vi "HTML Hierarhy Add Leaf.vi"(8 "error in":errorcluster, 10 "id":string, 11 "label":string) -> (0 "error out":errorcluster)   [LabVIEW 2014, in "lvprj2html.lvlib"]
uses:
  lvprj2html.lvlib
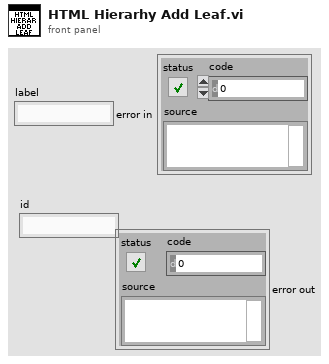
[diagram p1: front panel]
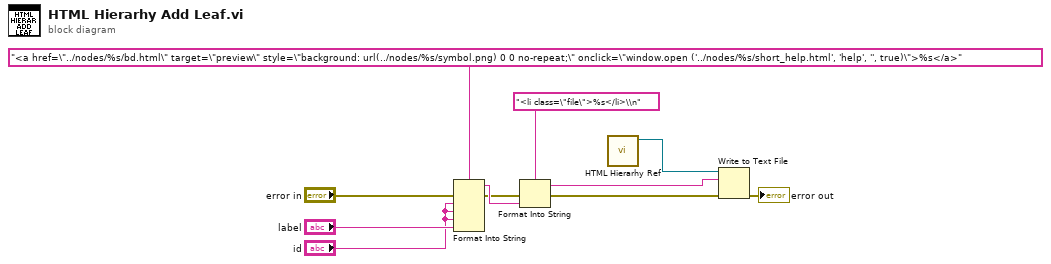
[diagram p0: block diagram]
diagram:
  n1 = Format Into String(format string="<a href=\"../nodes/%s/bd.html\" target=\"preview\" style=\"background: url(../nodes/%s/symbol.png) 0 0 no-repeat;\" onclick=\"window.open ('../nodes/%s/short_help.html', 'help', '', true)\">%s</a>" ("text"), error in="error in", "id", "id", "id", "label") -> (resulting string=w6:string, error out=w3:errorcluster)  [unwired: 1 in]
  n2 = Format Into String(format string="<li class=\"file\">%s</li>\\n" ("text"), error in=w3, w6) -> (resulting string=w5:string, error out=w2:errorcluster)  [unwired: 1 in]
  n3 = call "HTML Hierarhy Ref.vi"() -> ("Byte Stream File out"=w11:refnum<file>)  [unwired: 11 in]
  n4 = Write to Text File(file (use dialog)=w11, text=w5, error in=w2) -> (error out=→"error out":errorcluster)  [unwired: 1 in, 2 out]
